vi "ToFloat.vi"(1 "index":i32, 2 "array":u8[](array[numeric])) -> (0 "sp float":sgl)   [LabVIEW 2009]
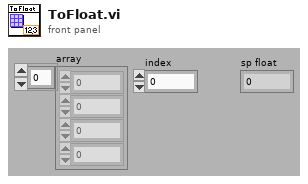
[diagram p1: front panel]
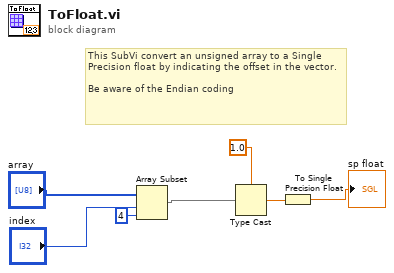
[diagram p0: block diagram]
diagram:
  # "This SubVi convert an unsigned array to a Single Precision float by indicating the offset in the vector.\n\nBe aware of the Endian coding"
  n1 = Array Subset(array="array", index="index", length=4) -> (w4:u8[])
  n2 = Type Cast(type=sgl 1.0 ("sp float"), x=w4) -> (*(type *) &x=w2:sgl)
  n3 = To Single Precision Float(number=w2) -> (single precision float=→"sp float":sgl)
